vi "Start.vi"(8 "error in (no error)":errorcluster, 11 "WaveformTask in":refnum<class "WaveformTask.lvclass">) -> (0 "error out":errorcluster, 3 "WaveformTask out":refnum<class "WaveformTask.lvclass">)   [LabVIEW 2015, in "WaveformTask.lvclass"]
uses:
  WaveformTask.lvclass
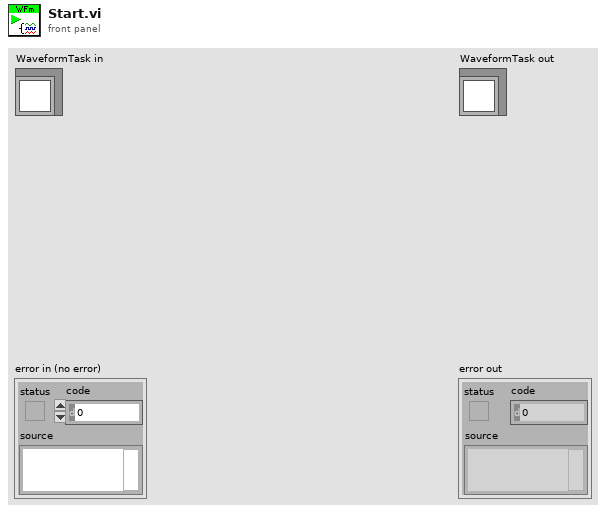
[diagram p1: front panel]
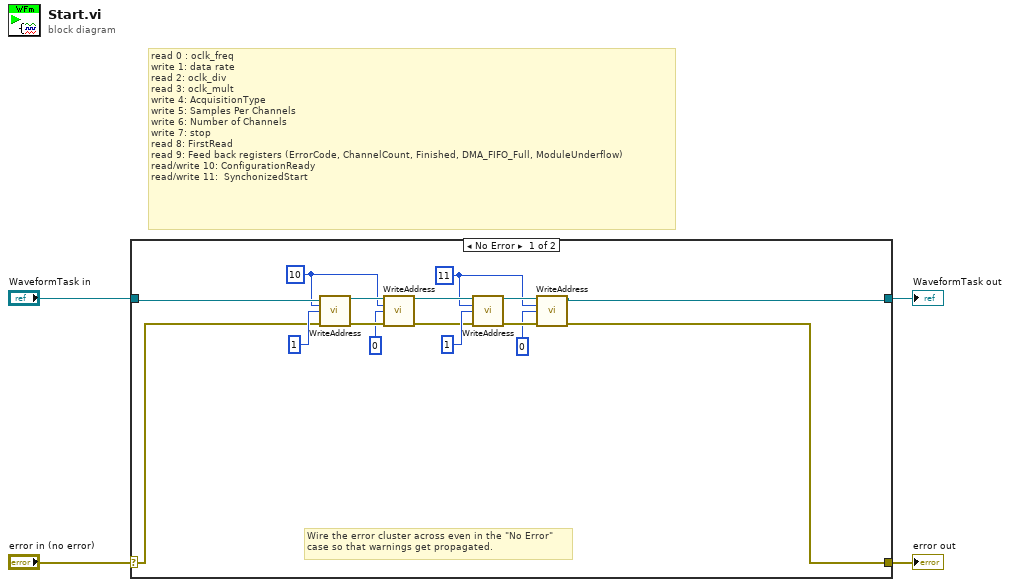
[diagram p0: block diagram]
diagram:
  # "read 0 : oclk_freq\nwrite 1: data rate\nread 2: oclk_div\nread 3: oclk_mult\nwrite 4: AcquisitionType\nwrite 5: Samples Per Channels\nwrite 6: Number of Channels\nwrite 7: stop\nread 8: FirstRead\nread 9: Feed back registers (ErrorCode, ChannelCount, Finished, DMA_FIFO_Full, ModuleUnderflow)\nread/write 10: ConfigurationReady\nread/write 11:  SynchonizedStart"
  n1 = case shown="No Error" "error in (no error)" {
    selector: "error in (no error)" -> [w9 w22]
    tunnel: [w5 w22] -> w3
    tunnel: [w6 w21] -> w1
    tunnel: "WaveformTask in" -> [w8 w21]
    frame No Error {
      w7 = u64 10 ("address")
      w10 = u64 11 ("address")
      # "Wire the error cluster across even in the \"No Error\"\ncase so that warnings get propagated."
      n2 = call "WriteAddress.vi"("Task in"=w8, "address"=w7, "data"=u64 1, "error in (no error)"=w9) -> ("Task out"=w19:refnum<class "WaveformTask.lvclass">, "error out"=w18:errorcluster)  [unwired: 10 in]
      n3 = call "WriteAddress.vi"("Task in"=w19, "address"=w7, "data"=u64 0, "error in (no error)"=w18) -> ("Task out"=w12:refnum<class "WaveformTask.lvclass">, "error out"=w11:errorcluster)  [unwired: 10 in]
      n4 = call "WriteAddress.vi"("Task in"=w12, "address"=w10, "data"=u64 1, "error in (no error)"=w11) -> ("Task out"=w15:refnum<class "WaveformTask.lvclass">, "error out"=w14:errorcluster)  [unwired: 10 in]
      n5 = call "WriteAddress.vi"("Task in"=w15, "address"=w10, "data"=u64 0, "error in (no error)"=w14) -> ("Task out"=w6:refnum<class "WaveformTask.lvclass">, "error out"=w5:errorcluster)  [unwired: 10 in]
    }
    frame Error {
    }
  }
  "error out" <- w3
  "WaveformTask out" <- w1
